vi "FTW-Actor-InboxAddress-Get.vi"(8 "error in (no error)":errorcluster, 11 "FTW-ActorInstance in":refnum<class "FTW-ActorInstance.lvclass">) -> (0 "error out":errorcluster, 2 "Inbox Address":string, 3 "FTW-ActorInstance out":refnum<class "FTW-ActorInstance.lvclass">)   [LabVIEW 2012, in "FTW-Actor.lvlib" / "FTW-ActorInstance.lvclass"]
uses:
  FTW-ActorInstance.lvclass
  FTW-ActorInstance.lvclass/FTW-ActorInstance.ctl
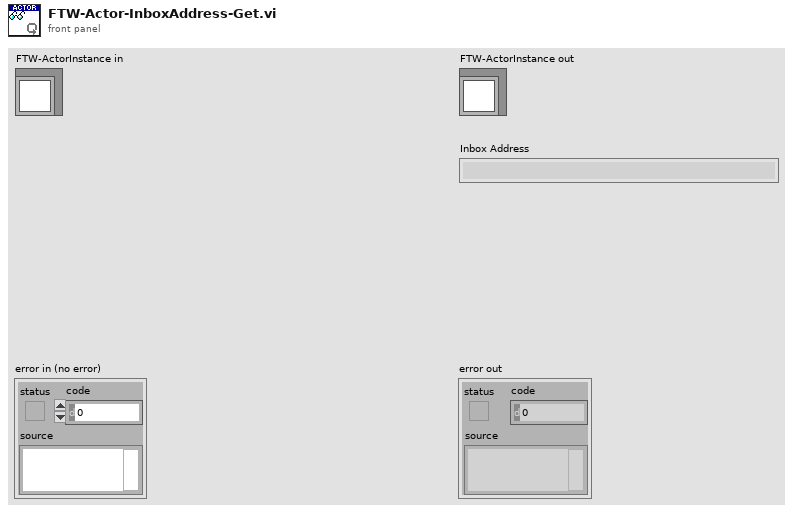
[diagram p1: front panel]
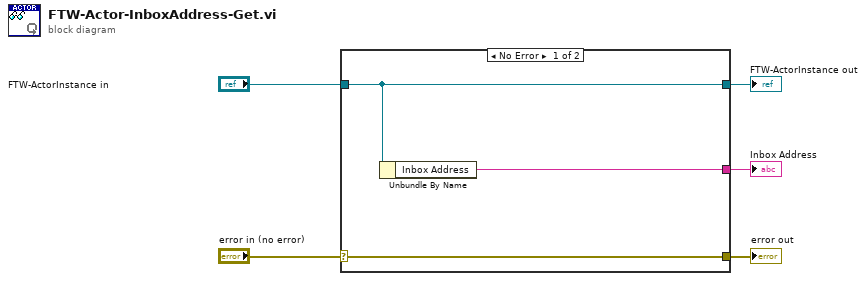
[diagram p0: block diagram]
diagram:
  n1 = case shown="No Error" "error in (no error)" {
    selector: "error in (no error)" -> [w8 w9]
    tunnel: [w8 w9] -> w4
    tunnel: [w7 w10] -> w2
    tunnel: "FTW-ActorInstance in" -> [w7 w10]
    tunnel: [w6 _] -> w1
    frame No Error {
      n2 = Unbundle By Name(w7) -> ("Inbox Address"=w6:string)
    }
    frame Error {
    }
  }
  "error out" <- w4
  "FTW-ActorInstance out" <- w2
  "Inbox Address" <- w1
